vi "ex4_3.vi"() -> ()   [LabVIEW 2020]
panel:
  in  "N":i32
  out "Out 1":dbl[][](array[numeric])
  in  "M":i32
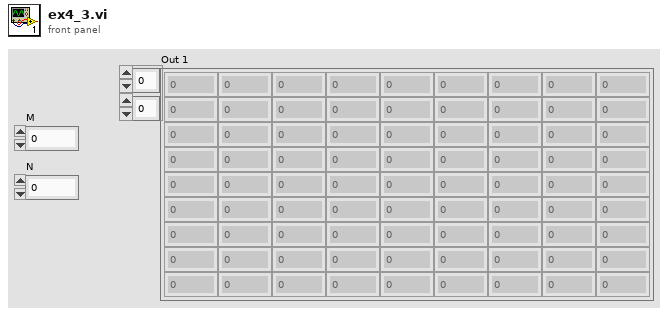
[diagram p1: front panel]
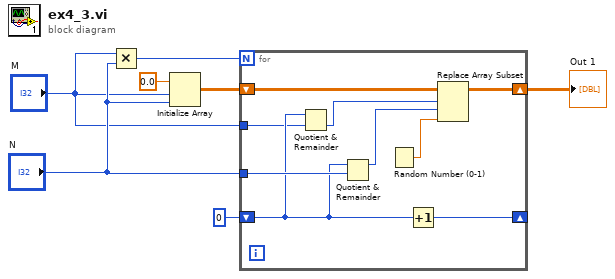
[diagram p0: block diagram]
diagram:
  n1 = Multiply(x="M", y="N") -> (x*y=w2:i32)
  n2 = Initialize Array(0.0, "M", "N") -> (w6:dbl[][])
  n3 = for {
    N: w2 -> [_]
    shift-right: [w15] -> w4
    shift-left: w6 -> [w16]
    shift-right: [w14] -> _
    shift-left: 0 -> [w12]
    tunnel: "N" -> [w13]
    tunnel: "M" -> [w8]
    n4 = Quotient & Remainder(x=w12, y=w8) -> (floor(x/y)=w10:i32)  [unwired: 1 out]
    n5 = Quotient & Remainder(x=w12, y=w13) -> (x-y*floor(x/y)=w9:i32)  [unwired: 1 out]
    n6 = Random Number (0-1)() -> (number: 0 to 1=w11:dbl)
    n7 = Increment(x=w12) -> (x+1=w14:i32)
    n8 = Replace Array Subset(array=w16, new element=w11, index (row)=w10, index (col)=w9) -> (w15:dbl[][])
  }
  "Out 1" <- w4
